vi "FF_GetForceComponents.vi"(8 "error in (no error)":errorcluster, 11 "Force Field Controller in":refnum<class "ForceField.lvclass">) -> (0 "error out":errorcluster, 2 "Force Component":dbl[](array[numeric]), 3 "Force Field Controller out":refnum<class "ForceField.lvclass">)   [LabVIEW 2015, in "ForceField.lvclass"]
uses:
  ForceField.lvclass
  ForceField.lvclass/ForceField.ctl
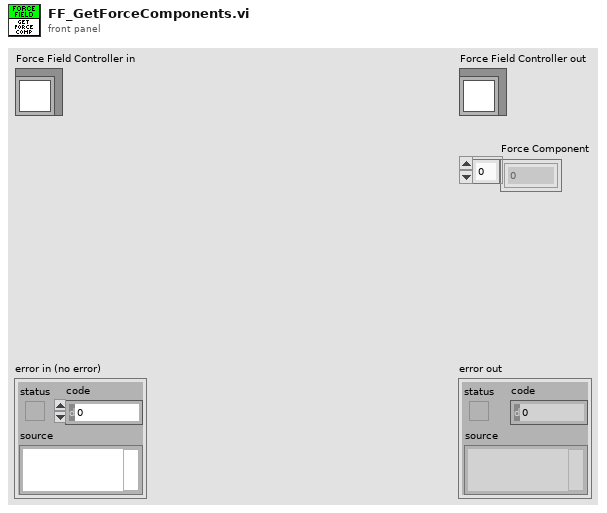
[diagram p1: front panel]
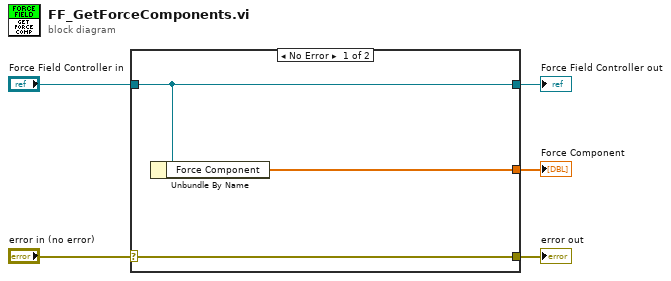
[diagram p0: block diagram]
diagram:
  n1 = case shown="No Error" "error in (no error)" {
    selector: "error in (no error)" -> [w8 w9]
    tunnel: [w8 w9] -> w4
    tunnel: [w7 w10] -> w2
    tunnel: "Force Field Controller in" -> [w7 w10]
    tunnel: [w6 _] -> w1
    frame No Error {
      n2 = Unbundle By Name(w7) -> ("Force Component"=w6:dbl[])
    }
    frame Error {
    }
  }
  "error out" <- w4
  "Force Field Controller out" <- w2
  "Force Component" <- w1
